vi "acquisitionHMSfromS.vi"(0 "seconds":i32) -> (1 "hours":i32, 2 "minutes":i32, 3 "seconds":i32, 4 "formatted string":string)   [LabVIEW 2017]
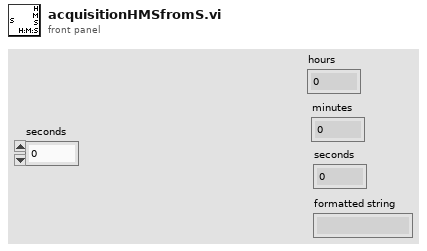
[diagram p1: front panel]
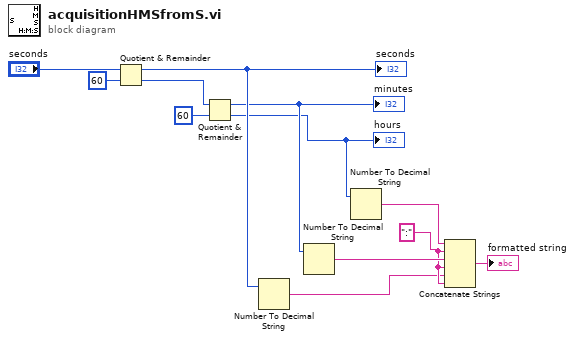
[diagram p0: block diagram]
diagram:
  w3 = ":" ("string")
  n1 = Quotient & Remainder(x="seconds", y=60) -> (x-y*floor(x/y)=w8:i32, floor(x/y)=w10:i32)
  "seconds" <- w8
  n2 = Quotient & Remainder(x=w10, y=60) -> (x-y*floor(x/y)=w7:i32, floor(x/y)=w6:i32)
  "minutes" <- w7
  "hours" <- w6
  n3 = Number To Decimal String(number=w8) -> (decimal integer string=w2:string)  [unwired: 1 in]
  n4 = Number To Decimal String(number=w7) -> (decimal integer string=w4:string)  [unwired: 1 in]
  n5 = Number To Decimal String(number=w6) -> (decimal integer string=w5:string)  [unwired: 1 in]
  n6 = Concatenate Strings(w5, w3, w4, w3, w2, w3) -> (→"formatted string":string)
